vi "Kalman filter_subvi.vi"(6 "Previous predicted pixel value":fxp<+,32,16>, 7 "Kalman gain":fxp<+,16,1>=0.1015625, 8 "Frame number":u16, 9 "Filter gain":fxp<+,16,0>=0.8000030517578125, 10 "Pixel value":u16, 11 "Input valid":bool=TRUE) -> (0 "Kalman filter result":fxp<+/-,36,20>, 3 "output valid":bool)   [LabVIEW 2015]
uses:
  <vilib>/Platform/TimedLoop/XDataNode/timing_clust.ctl
  <vilib>/Platform/TimedLoop/XDataNode/nitl_modes.ctl
  <vilib>/Platform/TimedLoop/XDataNode/wakeup.ctl
  <vilib>/rvi/Emulation/niFpgaSctlEmulationGetInTimedLoop.vi
  <vilib>/rvi/Emulation/niFpgaEmulationReportErrorSimple.vi
  <vilib>/rvi/Emulation/niFpgaGetClockAttributes.vi
  <vilib>/rvi/Emulation/niFpgaCriticalErrorInLSC.vi
  <vilib>/Platform/TimedLoop/XDataNode/XDataNode.xnode
  <vilib>/rvi/FXPMathLib/FxpSub/XNode/nifxpmath_Sub.xnode
  <vilib>/rvi/FXPMathLib/FxpMul/XNode/nifxpmath_Multiplier.xnode
  <vilib>/rvi/FXPMathLib/FxpAdd/XNode/nifxpmath_Add.xnode
  <vilib>/rvi/FXPMathLib/sim/FxpSim.dll
  <vilib>/Platform/TimedLoop/XDataNode/XDNodeRunTimeDep.lvlib
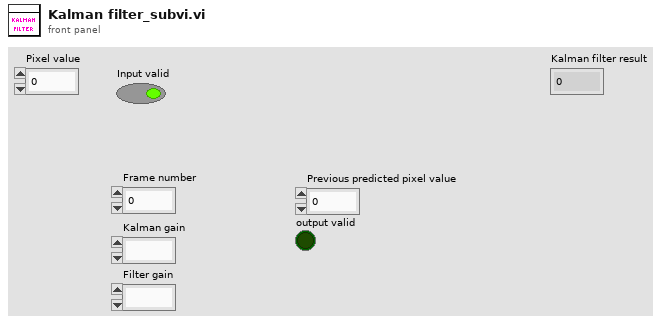
[diagram p1: front panel]
types:
  T1 = typedef "XDNodeRunTimeDep.lvlib/timing_clust.ctl" = cluster{"Expected End [f-1]":u64, "Actual End [f-1]":u64, "Finished Late? [f-1]":bool, "Expected End [i-1]":u64, "Actual End [i-1]":u64, "Finished Late? [i-1]":bool, "Expected Start [i]":u64, "Actual Start [i]":u64, "Expected Start [f]":u64, "Actual Start [f]":u64, "Source Name":string, "Structure Name":string, "Period":i64, "Deadline":i64, "Offset":i64, "Start":i64, "Priority":i32, "Timeout":i32, "Mode":T2, "Wakeup Reason":T3, "Error":errorcluster, "Source Type":string, "Secondary Source Type":string, "Global End Time":u64, "Global Start Time":u64, "Frame Duration":u64, "Iteration Duration":u64, "Assigned CPU":i32, "I/O Scan Engine Mode":u32}
  T2 = typedef "XDNodeRunTimeDep.lvlib/nitl_modes.ctl" = enum32{"No Change", "Process missed periods, maintain original phase", "Discard missed periods, maintain original phase", "Process missed periods, ignore original phase", "Discard missed periods, ignore original phase"}
  T3 = typedef "XDNodeRunTimeDep.lvlib/wakeup.ctl" = enum32{"Normal", "Aborted", "Asynchronous wakeup", "Timing source error", "Timed loop error", "Timeout"}
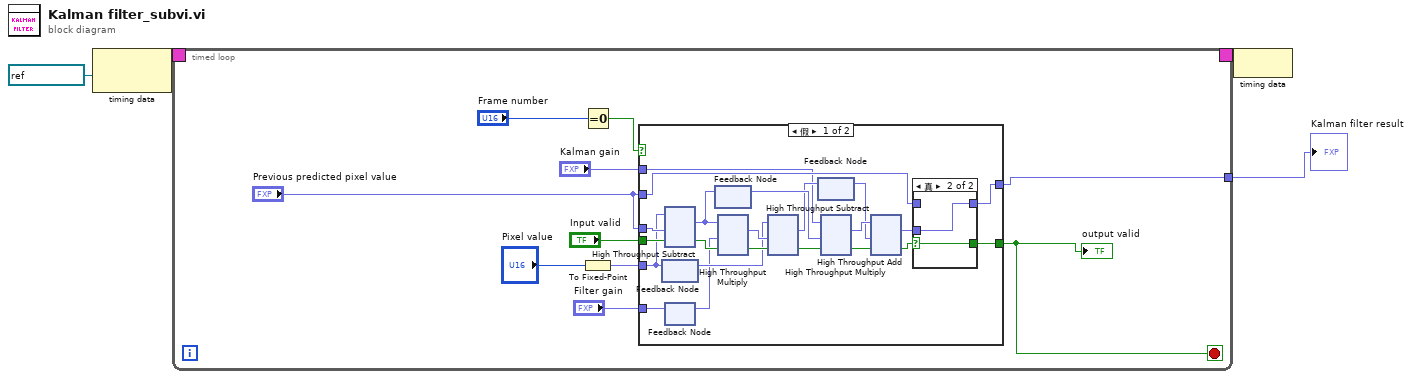
[diagram p0: block diagram]
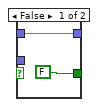
[diagram p2: hidden frame]
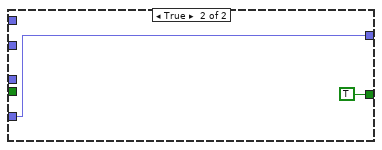
[diagram p3: hidden frame]
diagram:
  n1 = node-c288(refnum<k21> "200MHz" ("Source Name")) -> (w4:T1)
  n2 = timed-loop {
    timing: w4 -> [_]
    timing-out: [_] -> w3
    tunnel: [w5] -> w1
    stop <- w6 stop-if-true
    n3 = Equal To 0?(x="Frame number") -> (x = 0?=w11:bool)
    n4 = To Fixed-Point(number="Pixel value") -> (fixed-point=w7:fxp<+,16,16>)  [unwired: 1 in]
    n5 = case shown="假" w11 {
      tunnel: "Kalman gain" -> [w16 _]
      tunnel: w7 -> [w22 w42]
      tunnel: [w17 w42] -> w5
      tunnel: "Previous predicted pixel value" -> [w36 _]
      tunnel: "Input valid" -> [w35 _]
      tunnel: "Filter gain" -> [w20 _]
      tunnel: [w24 TRUE] -> w6
      tunnel: "Previous predicted pixel value" -> [w23 _]
      frame False {
        n6 = feedback #1() -> (w21:fxp<+,16,16>)  [unwired: 1 in]
        n7 = feedback-in #1(w22) -> ()
        n8 = xnode "High Throughput Subtract"("x"=w22, "y"=w36, "输入有效"=w35) -> ("x-y"=w29:fxp<+/-,34,18>, "输出有效"=w34:bool)  [unwired: 1 in, 1 out]
        n9 = feedback #2() -> (w19:fxp<+,16,0>)  [unwired: 1 in]
        n10 = feedback-in #2(w20) -> ()
        n11 = feedback #3() -> (w28:fxp<+/-,34,18>)  [unwired: 1 in]
        n12 = feedback-in #3(w29) -> ()
        n13 = xnode ("High Throughput Multiply")("x"=w29, "y"=w19, "输入有效"=w34) -> ("x*y"=w33:fxp<+/-,50,18>, "输出有效"=w32:bool)  [unwired: 1 in, 1 out]
        n14 = xnode "High Throughput Subtract"("x"=w21, "y"=w33, "输入有效"=w32) -> ("x-y"=w27:fxp<+/-,51,19>, "输出有效"=w18:bool)  [unwired: 1 in, 1 out]
        n15 = feedback #4() -> (w26:fxp<+/-,51,19>)  [unwired: 1 in]
        n16 = feedback-in #4(w27) -> ()
        n17 = xnode ("High Throughput Multiply")("x"=w16, "y"=w28, "输入有效"=w18) -> ("x*y"=w31:fxp<+/-,50,19>, "输出有效"=w30:bool)  [unwired: 1 in, 1 out]
        n18 = xnode ("High Throughput Add")("x"=w31, "y"=w26, "输入有效"=w30) -> ("x+y"=w25:fxp<+/-,32,20>, "输出有效"=w15:bool)  [unwired: 1 in, 1 out]
        n19 = case shown="真" w15 {
          selector: w15 -> [_ w40]
          tunnel: w25 -> [_ w39]
          tunnel: [FALSE w40] -> w24
          tunnel: w23 -> [w37 _]
          tunnel: [w37 w39] -> w17
          frame False {
          }
          frame True {
          }
        }
      }
      frame True {
      }
    }
    "output valid" <- w6
  }
  "Kalman filter result" <- w1
  n20 = node-c288(w3) -> ()
